vi "Set nidaqmx_grpc_GetTaskAttributeStringRequest.vi"(7 "Complete Call (T)":bool=TRUE, 8 "error in (no error)":errorcluster, 10 "package_templatemessage":T1, 11 "gRPCid":T3) -> (0 "error out":errorcluster)   [LabVIEW 2021, in "NI DAQmx_server.lvlib"]
uses:
  NI DAQmx_server.lvlib
  <vilib>/gRPC/LabVIEW gRPC Library/Shared/grpcId.ctl
  nidaqmx_grpc_GetTaskAttributeStringRequest.ctl
  nidevice_grpc_Session_session/nidevice_grpc_Session_session.lvclass
  nidaqmx_grpc_GetTaskAttributeStringRequest_attribute_enum/nidaqmx_grpc_GetTaskAttributeStringRequest_attribute_enum.lvclass
  nidevice_grpc_Session.ctl
  nidaqmx_grpc_GetTaskAttributeStringRequest_Flat.ctl
  nidevice_grpc_Session_Flat.ctl
  nidaqmx_grpc_TaskStringAttribute.ctl
  nidevice_grpc_Session_session/nidevice_grpc_Session_session.lvclass/nidevice_grpc_Session_session.ctl
  nidaqmx_grpc_GetTaskAttributeStringRequest_attribute_enum/nidaqmx_grpc_GetTaskAttributeStringRequest_attribute_enum.lvclass/nidaqmx_grpc_GetTaskAttributeStringRequest_attribute_enum.ctl
  dcc74a39-081a-4bdd-860b-8ed792803c96.vi
  RichToFlatnidevice_grpc_Session.vi
  nidaqmx_grpc_GetTaskAttributeStringRequest_attribute_enum/GetActiveFieldIndex.vi
  nidaqmx_grpc_GetTaskAttributeStringRequest_attribute_enum/Getattribute.vi
  nidaqmx_grpc_GetTaskAttributeStringRequest_attribute_enum/Getattribute_raw.vi
  <vilib>/gRPC/LabVIEW gRPC Library/Shared/TranslateGrpcError.vi
  nidevice_grpc_Session_session/GetActiveFieldIndex.vi
  nidevice_grpc_Session_session/Getname.vi
  nidevice_grpc_Session_session/Getid.vi
  <vilib>/gRPC/LabVIEW gRPC Library/Server API/Server/Get Server DLL Path.vi
  <vilib>/Utility/error.llb/Error Cluster From Error Code.vi
  <vilib>/gRPC/LabVIEW gRPC Library/grpc-lvsupport-release.lvlib
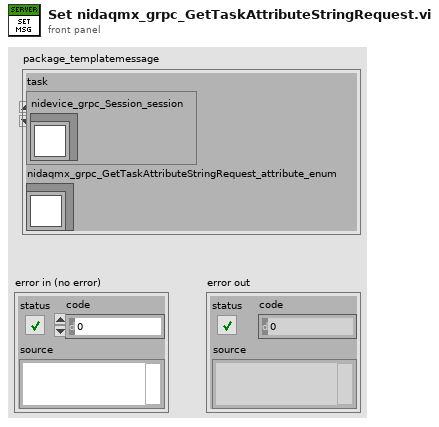
[diagram p1: front panel]
types:
  T1 = typedef "NI DAQmx_server.lvlib/nidaqmx_grpc_GetTaskAttributeStringRequest.ctl" = cluster{"task":T2, "nidaqmx_grpc_GetTaskAttributeStringRequest_attribute_enum":refnum<class "nidaqmx_grpc_GetTaskAttributeStringRequest_attribute_enum.lvclass">}
  T2 = typedef "NI DAQmx_server.lvlib/nidevice_grpc_Session.ctl" = cluster{"nidevice_grpc_Session_session":refnum<class "nidevice_grpc_Session_session.lvclass">}
  T3 = typedef "grpc-lvsupport-release.lvlib/grpcId.ctl" = u64
  T4 = typedef "NI DAQmx_server.lvlib/nidaqmx_grpc_GetTaskAttributeStringRequest_Flat.ctl" = cluster{"task":T5, "nidaqmx_grpc_GetTaskAttributeStringRequest_attribute_enum_selected_index":i32, "attribute":T6, "attribute_raw":i32}
  T5 = typedef "NI DAQmx_server.lvlib/nidevice_grpc_Session_Flat.ctl" = cluster{"nidevice_grpc_Session_session_selected_index":i32, "name":string, "id":u32}
  T6 = typedef "NI DAQmx_server.lvlib/nidaqmx_grpc_TaskStringAttribute.ctl" = enum32{"TASK_STRING_ATTRIBUTE_UNSPECIFIED", "TASK_ATTRIBUTE_CHANNELS", "TASK_ATTRIBUTE_NAME", "TASK_ATTRIBUTE_DEVICES"}
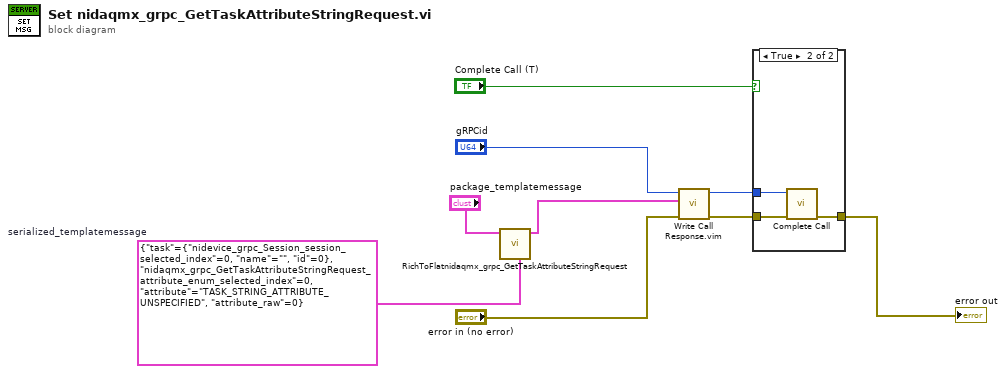
[diagram p0: block diagram]
diagram:
  w2 = T4 {"task"={"nidevice_grpc_Session_session_selected_index"=0, "name"="", "id"=0}, "nidaqmx_grpc_GetTaskAttributeStringRequest_attribute_enum_selected_index"=0, "attribute"=enum."TASK_STRING_ATTRIBUTE_UNSPECIFIED", "attribute_raw"=0}  # serialized_templatemessage
  n1 = call "RichToFlatnidaqmx_grpc_GetTaskAttributeStringRequest.vi"("OutputClusterType"=w2, "InputCluster"="package_templatemessage") -> ("OutputCluster"=w1:T4)  [unwired: 9 in]
  n2 = call "Write Call Response.vim"("error in"="error in (no error)", "Response Data"=w1, "gRPCid in"="gRPCid") -> ("error out"=w6:errorcluster, "gRPCid out"=w7:T3)  [unwired: 7 in]
  n3 = case shown="True" "Complete Call (T)" {
    tunnel: [w10 w13] -> w9
    tunnel: w7 -> [_ w12]
    tunnel: w6 -> [w10 w11]
    frame False {
    }
    frame True {
      n4 = call <vilib>:"Complete Call.vi"("gRPCid"=w12, "error in"=w11) -> ("error out"=w13:errorcluster)  [unwired: 8 in]
    }
  }
  "error out" <- w9
